vi "DAQ Signal conditioning.vi"(10 "Gain":dbl, 11 "data":dynamicdata(waveform)) -> (1 "FFT - (RMS)":dynamicdata(waveform), 2 "Dynamic Data":dynamicdata(waveform))   [LabVIEW 2016]
uses:
  <vilib>/express/express analysis/Spectral/Block/exnSpectralBlock spectral measurements RMS poly.vi
  <vilib>/express/express analysis/Spectral/Block/exnSpectralBlock spectral measurements RMS DDT.vi
  <vilib>/express/express analysis/Spectral/XNode/ExpressSpectralMeasurementsBlockNode.xnode
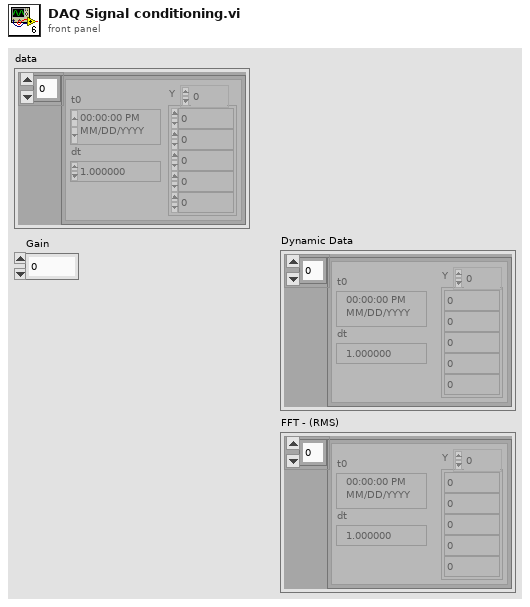
[diagram p1: front panel]
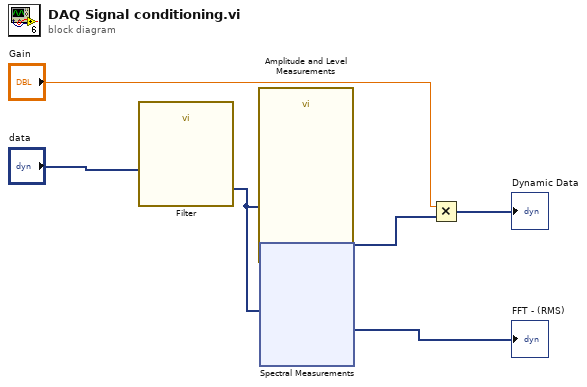
[diagram p0: block diagram]
diagram:
  n1 = call "Filter"("Signal"="data") -> ("Filtered Signal"=w6:dynamicdata)  [unwired: 9 in, 1 out]
  n2 = call "Amplitude and Level Measurements"("Signals"=w6) -> ("RMS"=w5:dynamicdata)  [unwired: 12 in, 2 out]
  n3 = xnode "Spectral Measurements"("信号"=w6) -> ("FFT - (RMS)"=→"FFT - (RMS)":dynamicdata)  [unwired: 1 in, 2 out]
  n4 = Multiply(x="Gain", y=w5) -> (x*y=→"Dynamic Data":dynamicdata)
